vi "LvMPDC_CMD_currentsong.vi"(6 "timeout_ms":i32=25000, 8 "error in (no error)":errorcluster, 9 "ReadBytes":i32=1024, 11 "Connect ID":refnum<k5>) -> (0 "error out":errorcluster, 1 "currentsong":T1 {"time" format="%<%H:%M:%S%3u>t"}, 3 "Connect ID out":refnum<k5>)   [LabVIEW 2012]
uses:
  LvMPDC_Typdef_currentsong.ctl
panel:
  # "LvMPDC:: CMD currentsong"
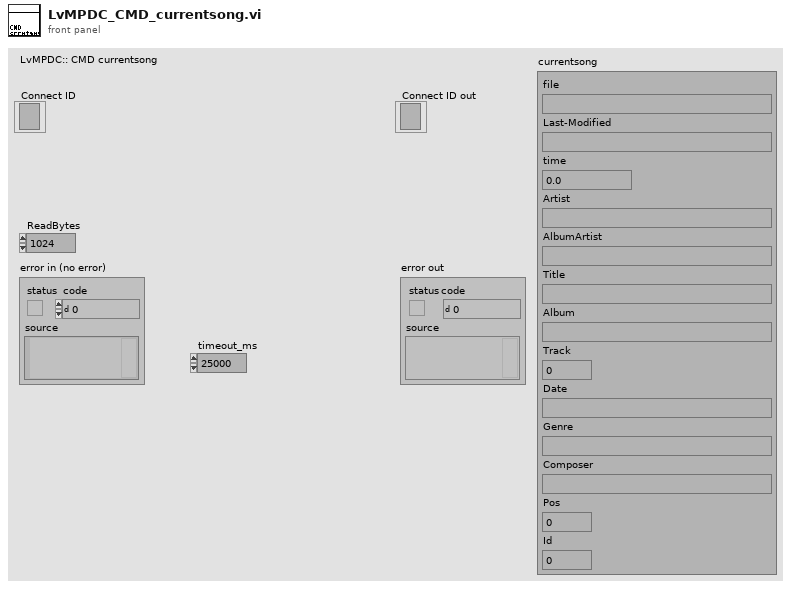
[diagram p1: front panel]
types:
  T1 = typedef "LvMPDC_Typdef_currentsong.ctl" = cluster{"file":path, "Last-Modified":string, "time":dbl, "Artist":string, "AlbumArtist":string, "Title":string, "Album":string, "Track":i32, "Date":string, "Genre":string, "Composer":string, "Pos":i32, "Id":i32}
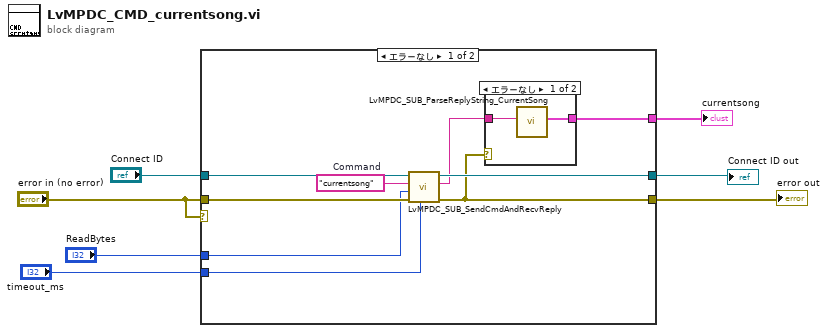
[diagram p0: block diagram]
diagram:
  n1 = case shown="エラーなし" "error in (no error)" {
    tunnel: "Connect ID" -> [w15 w20]
    tunnel: "error in (no error)" -> [w16 w19]
    tunnel: [w14 w20] -> w6
    tunnel: [w10 w19] -> w5
    tunnel: "timeout_ms" -> [w11 _]
    tunnel: "ReadBytes" -> [w12 _]
    tunnel: [w8 _] -> w1
    frame No Error {
      w13 = "currentsong"  # Command
      n2 = call "LvMPDC_SUB_SendCmdAndRecvReply.vi"("timeout_ms"=w11, "error in (no error)"=w16, "ReadBytes"=w12, "Command"=w13, "Connect ID"=w15) -> ("error out"=w10:errorcluster, "Reply"=w9:string, "Connect ID out"=w14:refnum<k5>)  [unwired: 4 in]
      n3 = case shown="エラーなし" w10 {
        tunnel: w9 -> [w18 _]
        tunnel: [w17 _] -> w8
        frame No Error {
          n4 = call "LvMPDC_SUB_ParseReplyString_CurrentSong.vi"("status reply string"=w18) -> ("currentsong"=w17:T1)  [unwired: 10 in]
        }
        frame Error {
        }
      }
    }
    frame Error {
    }
  }
  "Connect ID out" <- w6
  "error out" <- w5
  "currentsong" <- w1
